vi "setRelativeDisp.vi"(2 "disp":sgl, 3 "ID":i32, 4 "handle":i32, 5 "错误输入（无错误）":errorcluster) -> (0 "return":i32, 1 "错误输出":errorcluster)   [LabVIEW 2013, in "EM_CVx.lvlib"]
uses:
  EM_CVx.lvlib
  library/moverLibrary_x86.dll
  library/moverLibrary_x64.dll
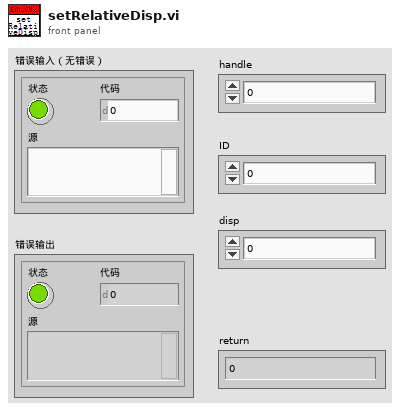
[diagram p1: front panel]
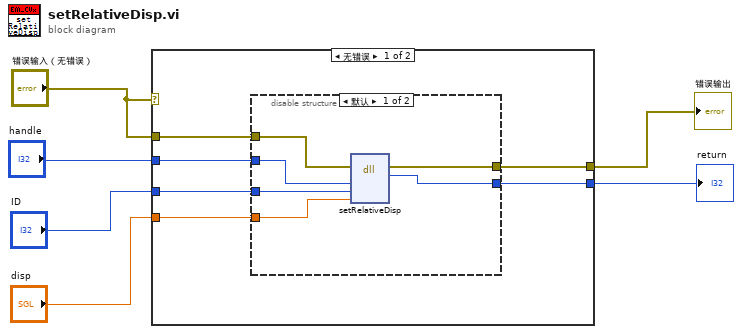
[diagram p0: block diagram]
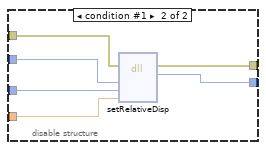
[diagram p2: hidden frame]
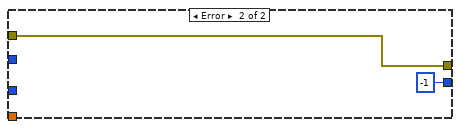
[diagram p3: hidden frame]
diagram:
  n1 = case shown="无错误" "错误输入（无错误）" {
    tunnel: "handle" -> [w12 _]
    tunnel: "ID" -> [w11 _]
    tunnel: "disp" -> [w10 _]
    tunnel: "错误输入（无错误）" -> [w9 w26]
    tunnel: [w8 -1 ("return")] -> w3
    tunnel: [w7 w26] -> w2
    frame No Error {
      n2 = disable-structure shown="默认" {
        disable-tunnel: w12 -> [w18 w21]
        disable-tunnel: w11 -> [w17 w22]
        disable-tunnel: w10 -> [w16 w23]
        disable-tunnel: w9 -> [w15 w20]
        disable-tunnel: [w14 w24] -> w8
        disable-tunnel: [w13 w19] -> w7
        frame condition #0 (active) {
          n3 = dll-call lib="E:/5-mover/4-labView/EM_CVx_2013/library/moverLibrary_x86.dll" fn="setRelativeDisp"(error in=w15, "handle"=w18, "ID"=w17, "disp"=w16) -> (error out=w13:errorcluster, "return"=w14:i32)  [unwired: 5 in, 1 out]
        }
        frame condition #1 {
          n4 = dll-call lib="E:/5-mover/4-labView/EM_CVx_2013/library/moverLibrary_x64.dll" fn="setRelativeDisp"(error in=w20, "handle"=w21, "ID"=w22, "disp"=w23) -> (error out=w19:errorcluster, "return"=w24:i32)  [unwired: 5 in, 1 out]
        }
      }
    }
    frame Error {
    }
  }
  "错误输出" <- w2
  "return" <- w3
